vi "Login.vi"(10 "窗口边界":T1) -> (0 "drop?":bool, 2 "User Name":string, 3 "User IP":string)   [LabVIEW 2014]
uses:
  <vilib>/Utility/miscctls.llb/LVRectTypeDef.ctl
panel:
  in  "Cancel":bool
  in  "OK":bool
  in  "Name":string="杭州立佳"
  in  "服务器 IP 地址":string="localhost"
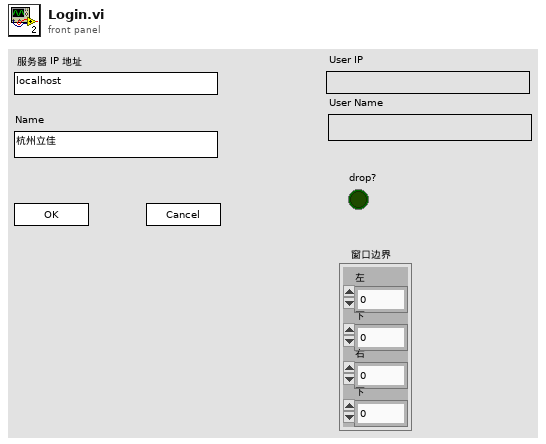
[diagram p1: front panel]
types:
  T1 = typedef "LVRectTypeDef.ctl" = cluster{"Left":i16, "Top":i16, "Right":i16, "Bottom":i16}
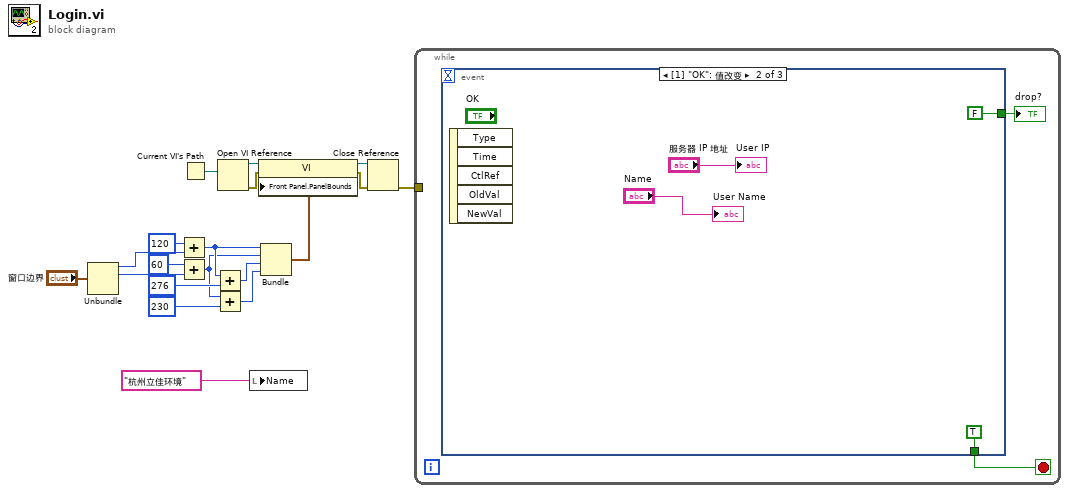
[diagram p0: block diagram]
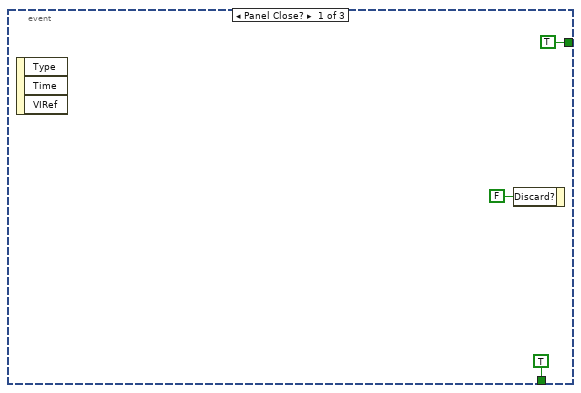
[diagram p2: hidden frame]
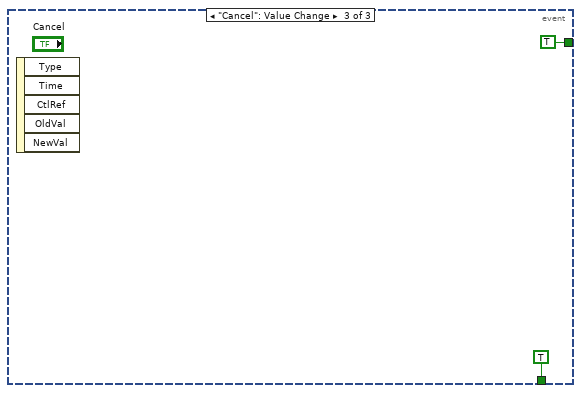
[diagram p3: hidden frame]
diagram:
  n1 = Unbundle("窗口边界") -> ("Left"=w11:i16, "Top"=w9:i16)  [unwired: 2 out]
  n2 = Add(x=i16 120, y=w11) -> (x+y=w6:i16)
  n3 = Add(x=i16 60, y=w9) -> (x+y=w5:i16)
  n4 = Current VI's Path() -> (path=w19:path)
  n5 = Add(x=w6, y=i16 276) -> (x+y=w4:i16)
  n6 = Add(x=w5, y=i16 230) -> (x+y=w3:i16)
  n7 = Open VI Reference(vi path=w19) -> (vi reference=w18:refnum<vi>, error out=w17:errorcluster)  [unwired: 5 in]
  n8 = local write "Name"("杭州立佳环境") -> ()
  n9 = Bundle(w6, w5, w4, w3) -> (w2:cluster{i16, i16, i16, i16})  [unwired: 1 in]
  n10 = property class="VI"(reference=w18, error in=w17, "Front Panel.PanelBounds"=w2) -> (reference out=w15:refnum<vi>, error out=w16:errorcluster)
  n11 = Close Reference(reference=w15, error in (no error)=w16) -> (error out=w14:errorcluster)
  n12 = while {
    tunnel: w14 -> [_]
    stop <- w20 stop-if-true
    n13 = event shown="[1] \"OK\": 值改变" {
      selector: _ -> [_ _ _]
      dyn-events: _ -> [_ _ _]
      timeout: _ -> [_ _ _]
      tunnel: [TRUE FALSE TRUE] -> w21
      tunnel: [TRUE TRUE TRUE] -> w20
      event Panel Close? {
        n14 = event-data() -> ()  [unwired: 1 in, 3 out]
        n15 = event-data("Discard?"=FALSE ("放弃？")) -> ()  [unwired: 1 in, 1 out]
      }
      event "OK": Value Change {
        n16 = event-data() -> ()  [unwired: 1 in, 5 out]
        "User IP" <- "服务器 IP 地址"
        "User Name" <- "Name"
      }
      event "Cancel": Value Change {
        n17 = event-data() -> ()  [unwired: 1 in, 5 out]
      }
    }
    "drop?" <- w21
  }
